vi "array tests.vi"() -> ()   [LabVIEW 2013, in "EthernetIP tests.lvlib"]
uses:
  EthernetIP tests.lvlib
  configuration/EthernetIP configuration.lvclass
  execution/EthernetIP runtime.lvclass
  configuration/assembly type.ctl
  <vilib>/NI/Tag Bus/tag/Data Type.ctl
  <vilib>/NI/Tag Bus/dictionary/data dictionary.lvclass/data dictionary.ctl
  <vilib>/NI/Tag Bus/dictionary/lookup polymorphs/locate Array of I16.vi
  <vilib>/NI/Tag Bus/table/data polymorphs/write one/write Array of I16.vi
  <vilib>/NI/Tag Bus/table/data polymorphs/read one/read Array of I16.vi
  <vilib>/NI/Tag Bus/dictionary/search/find data index.vi
  <vilib>/NI/Tag Bus/dictionary/search/search string list.vi
  <vilib>/NI/Tag Bus/dictionary/tag not found.vi
  <vilib>/NI/Tag Bus/tag/tag descriptor.lvclass
  <vilib>/NI/Tag Bus/dictionary/data dictionary.lvclass
  <vilib>/NI/Tag Bus/table/data table.lvlib
  channel/EthernetIP Channel.lvclass
  <vilib>/NI/Configuration Framework/serializable configuration/NISE_CEF_serializable configuration.lvclass
panel:
  in  "out":i16[](array[numeric])
  out "in":i16[](array[numeric])
  in  "stop":bool
  out "final error":errorcluster
  out "output error":errorcluster
  out "input error":errorcluster
  out "output lookup error":errorcluster
  out "no data written":bool
  out "input lookup error":errorcluster
  out "init error":errorcluster
  out "correct execution settings":bool
  out "serialization problem":errorcluster
  out "invalid configuration":errorcluster
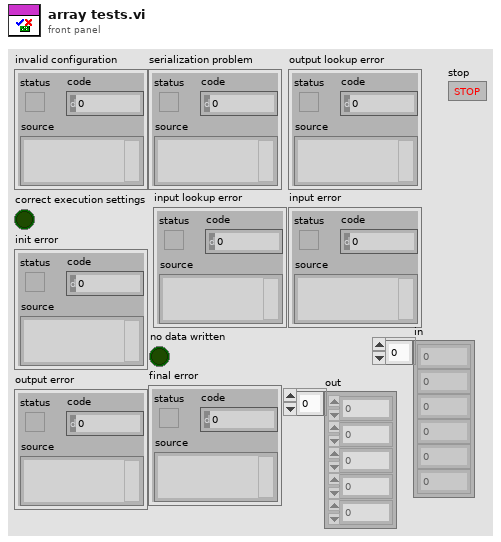
[diagram p1: front panel]
types:
  T1 = typedef "tag bus.lvlib/tag descriptor.lvclass/Data Type.ctl" = enum16{"Double", "Single", "I64", "I32", "I16", "I8", "U64", "U32", "U16", "U8", "Boolean", "String", "Array of Double", "Array of Single", "Array of I64", "Array of I32", "Array of I16", "Array of I8", "Array of U64", "Array of U32", "Array of U16", "Array of U8", "Array of Boolean", "Array of String"}
  T2 = typedef "EthernetIP configuration.lvclass/assembly type.ctl" = enum32{"Producing", "Consuming"}
  T3 = typedef "TBM channel.lvclass/data tables.ctl" = cluster{"input data":T4, "processing parameter":T4, "processing result":T4, "output data":T4}
  T4 = typedef "tag bus.lvlib/dictionary table pair.ctl" = cluster{"data dictionary":refnum<class "data dictionary.lvclass">, "data table":T5}
  T5 = typedef "tag bus.lvlib/data table.lvlib/data table.ctl" = cluster{"Double":dbl[], "Single":sgl[], "I64":i64[], "I32":i32[], "I16":i16[], "I8":i8[], "U64":u64[], "U32":u32[], "U16":u16[], "U8":u8[], "Boolean":bool[], "String":string[], "Array of Double":cluster{"DBL Array":dbl[]}[], "Array of Single":cluster{"SGL Array":sgl[]}[], "Array of I64":cluster{"I64 Array":i64[]}[], "Array of I32":cluster{"I32 Array":i32[]}[], "Array of I16":cluster{"I16 Array":i16[]}[], "Array of I8":cluster{"I8 Array":i8[]}[], "Array of U64":cluster{"U64 Array":u64[]}[], "Array of U32":cluster{"U32 Array":u32[]}[], "Array of U16":cluster{"U16 Array":u16[]}[], "Array of U8":cluster{"U8 Array":u8[]}[], "Array of Boolean":cluster{"Boolean Array":bool[]}[], "Array of String":cluster{"String Array":string[]}[]}
  T6 = typedef "TBM module execution interface.lvclass/execution settings.ctl" = cluster{"reads inputs":bool, "processes data":bool, "writes outputs":bool}
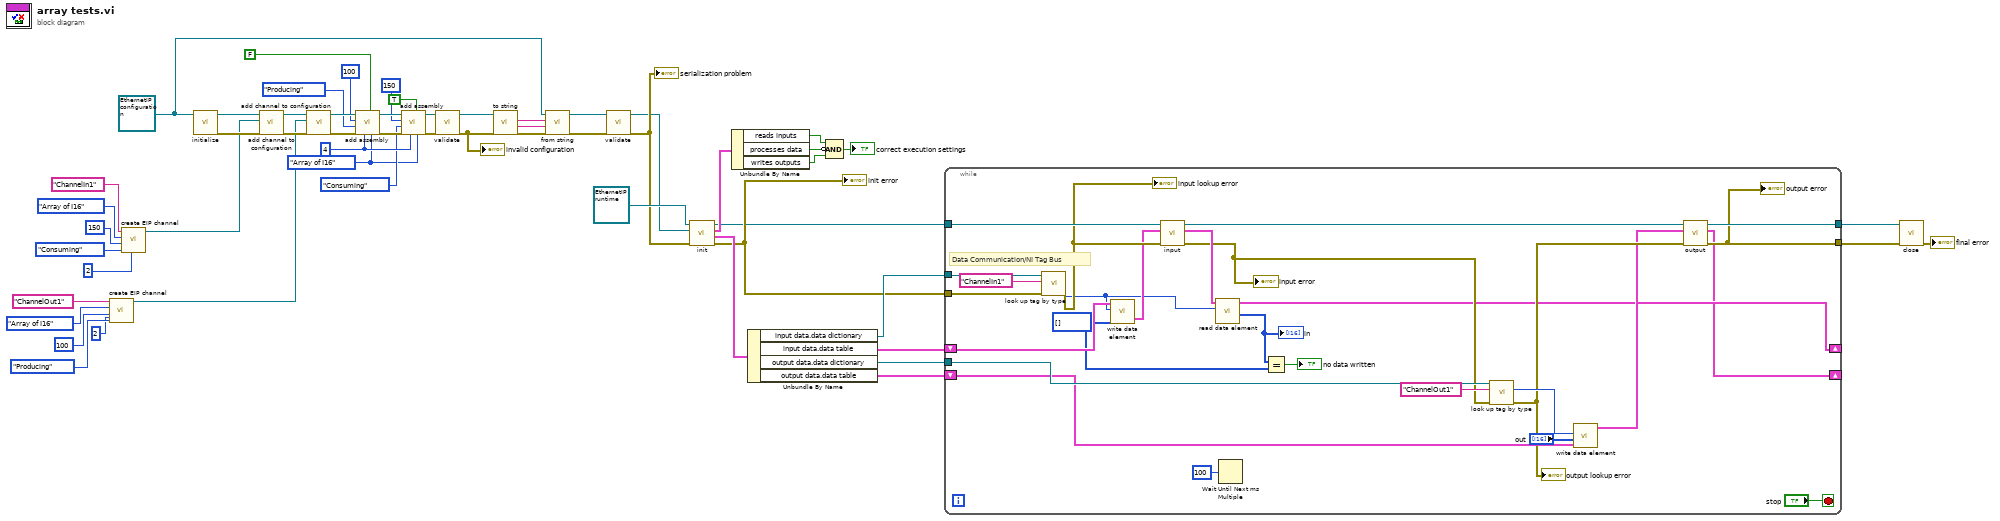
[diagram p0: block diagram]
diagram:
  w3 = Data_Type."Array of I16" ("data type")
  w9 = u32 4 ("Size (bytes)")
  w2 = refnum<class "EthernetIP configuration.lvclass"> refnum ("tag bus configurable plugin module configuration")
  n1 = call "create EIP channel.vi"("element"=2 ("byte index"), "Type"=assembly_type."Producing", "Instance ID"=u32 100, "data type"=Data_Type."Array of I16", "name"="ChannelOut1" ("channel name")) -> ("EthernetIP Channel out"=w20:refnum<class "EthernetIP Channel.lvclass">)  [unwired: 6 in]
  n2 = call "create EIP channel.vi"("element"=2 ("byte index"), "Type"=assembly_type."Consuming", "Instance ID"=u32 150, "data type"=Data_Type."Array of I16", "name"="ChannelIn1" ("channel name")) -> ("EthernetIP Channel out"=w14:refnum<class "EthernetIP Channel.lvclass">)  [unwired: 6 in]
  n3 = call <vilib>:"initialize.vi"("configuration in"=w2) -> ("error out"=w28:errorcluster, "configuration out"=w29:refnum<class "EthernetIP configuration.lvclass">)  [unwired: 8 in, 1 out]
  n4 = call "add channel to configuration.vi"("error in"=w28, "TBM channel in"=w14, "EthernetIP configuration in"=w29) -> ("error out"=w30:errorcluster, "EthernetIP configuration out"=w31:refnum<class "EthernetIP configuration.lvclass">)  [unwired: 7 in]
  n5 = call "add channel to configuration.vi"("error in"=w30, "TBM channel in"=w20, "EthernetIP configuration in"=w31) -> ("error out"=w27:errorcluster, "EthernetIP configuration out"=w12:refnum<class "EthernetIP configuration.lvclass">)  [unwired: 7 in]
  n6 = call "add assembly.vi"("data type"=w3, "big endian?"=FALSE, "size (elements)"=w9, "error in"=w27, "Type"=assembly_type."Producing", "instance ID"=u32 100 ("Instance ID"), "EthernetIP configuration in"=w12) -> ("error out"=w13:errorcluster, "EthernetIP configuration out"=w10:refnum<class "EthernetIP configuration.lvclass">)  [unwired: 3 in]
  n7 = call "add assembly.vi"("data type"=w3, "big endian?"=TRUE, "size (elements)"=w9, "error in"=w13, "Type"=assembly_type."Consuming", "instance ID"=u32 150 ("Instance ID"), "EthernetIP configuration in"=w10) -> ("error out"=w11:errorcluster, "EthernetIP configuration out"=w26:refnum<class "EthernetIP configuration.lvclass">)  [unwired: 3 in]
  n8 = call-dynamic "validate.vi"("error in"=w11, "EthernetIP configuration in"=w26) -> ("error out"=w55:errorcluster, "EthernetIP configuration out"=w56:refnum<class "EthernetIP configuration.lvclass">)  [unwired: 8 in]
  "invalid configuration" <- w55
  n9 = call-dynamic "to string.vi"("error in"=w55, "EthernetIP configuration in"=w56) -> ("error out"=w52:errorcluster, "data"=w53:string, "version"=w54:string)  [unwired: 6 in, 1 out]
  n10 = call-dynamic "from string.vi"("error in"=w52, "data"=w53, "version"=w54, "EthernetIP configuration in"=w2) -> ("error out"=w50:errorcluster, "EthernetIP configuration out"=w51:refnum<class "EthernetIP configuration.lvclass">)  [unwired: 6 in]
  n11 = call-dynamic "validate.vi"("error in"=w50, "EthernetIP configuration in"=w51) -> ("error out"=w48:errorcluster, "EthernetIP configuration out"=w47:refnum<class "EthernetIP configuration.lvclass">)  [unwired: 8 in]
  "serialization problem" <- w48
  n12 = call-dynamic "init.vi"("error in"=w48, "TBM module configuration in"=w47, "EthernetIP runtime in"=refnum<class "EthernetIP runtime.lvclass"> refnum ("tag bus configurable plugin module")) -> ("error out"=w39:errorcluster, "data allocations"=w41:T3, "execution settings"=w46:T6, "EthernetIP runtime out"=w37:refnum<class "EthernetIP runtime.lvclass">)  [unwired: 5 in]
  "init error" <- w39
  n13 = Unbundle By Name(w46) -> ("reads inputs"=w43:bool, "processes data"=w45:bool, "writes outputs"=w44:bool)
  n14 = Unbundle By Name(w41) -> ("input data.data dictionary"=w40:refnum<class "data dictionary.lvclass">, "input data.data table"=w38:T5, "output data.data dictionary"=w36:refnum<class "data dictionary.lvclass">, "output data.data table"=w35:T5)
  n15 = Compound Arithmetic op=AND(w43, invert w45, w44) -> (→"correct execution settings":bool)
  n16 = while {
    tunnel: w40 -> [w83]
    tunnel: w39 -> [w82]
    tunnel: w37 -> [w79]
    tunnel: w36 -> [w72]
    tunnel: [w64] -> w34
    tunnel: [w63] -> w33
    shift-right: [w61] -> _
    shift-left: w35 -> [w69]
    shift-right: [w62] -> _
    shift-left: w38 -> [w80]
    stop <- "stop" stop-if-true
    w58 = i16[] [] ("value")
    # "Data Communication/NI Tag Bus"
    n17 = call-poly <vilib>:"look up tag by type.vi"("error in"=w82, "name"="ChannelIn1" ("channel name"), "data dictionary in"=w83) -> ("error out"=w78:errorcluster, "index"=w75:i32)  [unwired: 6 in, 1 out]
    "input lookup error" <- w78
    n18 = call-poly <vilib>:"write data element.vi"("value"=w58, "index"=w75, "data table in"=w80) -> ("data table out"=w77:T5)  [unwired: 8 in]
    n19 = call-dynamic "input.vi"("error in"=w78, "data table in"=w77, "EthernetIP runtime in"=w79) -> ("error out"=w68:errorcluster, "data table out"=w76:T5, "EthernetIP runtime out"=w66:refnum<class "EthernetIP runtime.lvclass">)  [unwired: 6 in]
    "input error" <- w68
    n20 = call-poly <vilib>:"read data element.vi"("index"=w75, "data table in"=w76) -> ("value"=w74:i16[], "data table out"=w62:T5)  [unwired: 8 in]
    "in" <- w74
    n21 = Wait Until Next ms Multiple(millisecond multiple=u32 100) -> ()  [unwired: 1 out]
    n22 = Equal?(x=w74, y=w58) -> (x = y?=→"no data written":bool)
    n23 = call-poly <vilib>:"look up tag by type.vi"("error in"=w68, "name"="ChannelOut1" ("channel name"), "data dictionary in"=w72) -> ("error out"=w67:errorcluster, "index"=w70:i32)  [unwired: 6 in, 1 out]
    "output lookup error" <- w67
    n24 = call-poly <vilib>:"write data element.vi"("value"="out", "index"=w70, "data table in"=w69) -> ("data table out"=w65:T5)  [unwired: 8 in]
    n25 = call-dynamic "output.vi"("error in"=w67, "data table in"=w65, "EthernetIP runtime in"=w66) -> ("error out"=w63:errorcluster, "data table out"=w61:T5, "EthernetIP runtime out"=w64:refnum<class "EthernetIP runtime.lvclass">)  [unwired: 6 in]
    "output error" <- w63
  }
  n26 = call-dynamic "close.vi"("error in"=w33, "EthernetIP runtime in"=w34) -> ("error out"=→"final error":errorcluster)  [unwired: 9 in]
